vi "Transform And Project 1.vi"() -> ()   [LabVIEW 2022 SP3, in "Benchmark.lvlib"]
uses:
  Benchmark.lvlib
  3ca7c682-72f9-471a-94d6-f3f625e42330.vi
  717569c3-c8f8-4444-b08c-2f89a2934aa8.vi
  <vilib>/Utility/High Resolution Relative Seconds.vi
  <vilib>/Analysis/NI_AALBase.lvlib
panel:
  out "Histogram Graph":T1(graph)
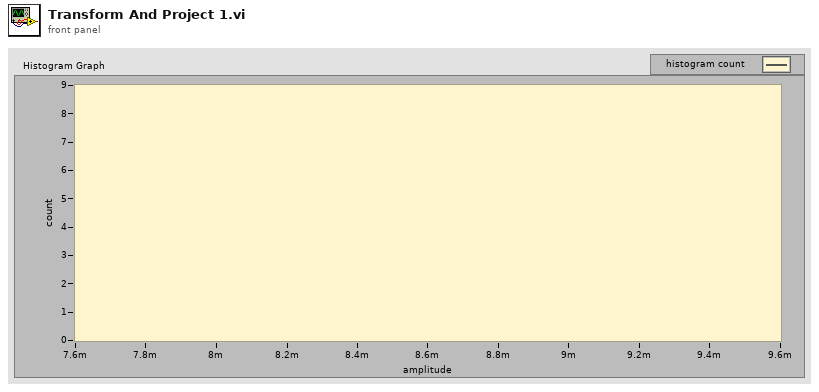
[diagram p1: front panel]
types:
  T1 = cluster{"X Values":dbl[], "Histogram: h(x)":i32[]}
  T2 = typedef "Core Data.ctl" = cluster{"Screen Dimensions":T3, "Camera":T4, "Transform":T5, "Line Colour":u32, "Fill Colour":u32, "Draw Lines":bool, "Projection Matrix":sgl[][], "Update Screen":bool, "Frame Buffer":refnum<data-value>, "Objects":T7[], "Camera Up":sgl, "Camera Left":sgl, "Camera Rotation":sgl, "Camera Forward":sgl, "Draw Triangles":bool, "Frame Buffer 2":refnum<data-value>, "Framebuffer":bool}
  T3 = typedef "Raster.lvlib/Screen Dimensions.ctl" = cluster{"Width":u32, "Height":u32}
  T4 = typedef "3D.lvlib/Camera.ctl" = cluster{"Field Of View":sgl, "Near Plane":sgl, "Far Plane":sgl}
  T5 = typedef "3D.lvlib/Transform.ctl" = cluster{"Position":T6, "Rotation":T6, "Scale":T6}
  T6 = typedef "3D.lvlib/Vector 3D.ctl" = cluster{"x":sgl, "y":sgl, "z":sgl}
  T7 = typedef "3D.lvlib/Mesh.ctl" = cluster{"Triangles":T8[]}
  T8 = typedef "3D.lvlib/Triangle 3D.ctl" = cluster{"Point 1":T6, "Point 2":T6, "Point 3":T6, "Fill Colour":u32}
  T9 = typedef "3D.lvlib/Triangle 2D.ctl" = cluster{"Point 1":T10, "Point 2":T10, "Point 3":T10, "Fill Colour":u32}
  T10 = typedef "3D.lvlib/Point 2D.ctl" = cluster{"x":sgl, "y":sgl}
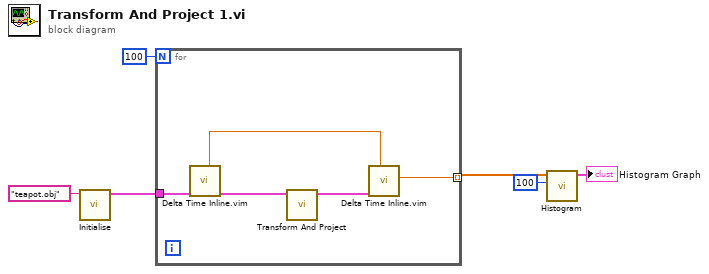
[diagram p0: block diagram]
diagram:
  n1 = call "Initialise.vi"("name or relative path"="teapot.obj") -> ("Core Data"=w2:T2)  [unwired: 9 in, 1 out]
  n2 = for {
    N: 100 -> [_]
    tunnel: w2 -> [w11]
    tunnel: [w7] -> w5 mode=indexing
    n3 = call "Delta Time Inline.vim"("value in"=w11) -> ("value out"=w10:T2, "Relative Seconds out [s]"=w8:dbl)  [unwired: 8 in, 1 out]
    n4 = call "Transform And Project.vi"("Core Data"=w10) -> ("Triangles Sorted"=w9:T9[])  [unwired: 9 in, 1 out]
    n5 = call "Delta Time Inline.vim"("Relative Seconds in [s]"=w8, "value in"=w9) -> ("Delta Time [s]"=w7:dbl)  [unwired: 7 in, 2 out]
  }
  n6 = call <vilib>:"Histogram.vi"("intervals"=100, "X"=w5) -> ("Histogram Graph"=→"Histogram Graph":T1)  [unwired: 6 in, 3 out]
